vi "toggle1-26-13.vi"(11 "input":bool) -> (3 "output":bool)   [LabVIEW 2015]
uses:
  <vilib>/ptbypt/NI_PtbyPt.lvlib
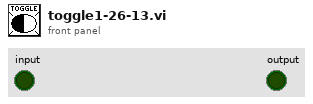
[diagram p1: front panel]
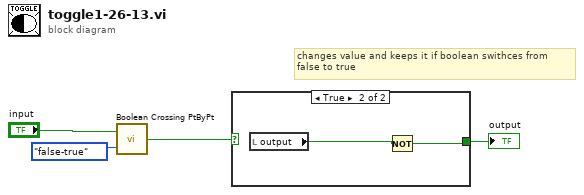
[diagram p0: block diagram]
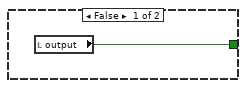
[diagram p2: hidden frame]
diagram:
  # "changes value and keeps it if boolean swithces from \nfalse to true"
  n1 = call <vilib>:"Boolean Crossing PtByPt.vi"("direction"=enum16{"either", "false-true", "true-false"}."false-true", "input"="input") -> ("crossing"=w1:bool)  [unwired: 1 in]
  n2 = case shown="True" w1 {
    tunnel: [w5 w6] -> w4
    frame False {
      n3 = local read "output"() -> (w5:bool)
    }
    frame True {
      n4 = local read "output"() -> (w7:bool)
      n5 = Not(x=w7) -> (.not. x?=w6:bool)
    }
  }
  "output" <- w4
